vi "Emitter.Test.vi"() -> ()   [LabVIEW 2016]
panel:
  in  "input json string":string="{\"values\":\"test\"}"
  in  "exchange name":u16(ring) items=["requests", "alerts"]
  in  "routing key":string="broadcast"
  out "error out":errorcluster
  in  "error (in)":errorcluster
  in  "host name":string="higgsino.physics.ucsb.edu"
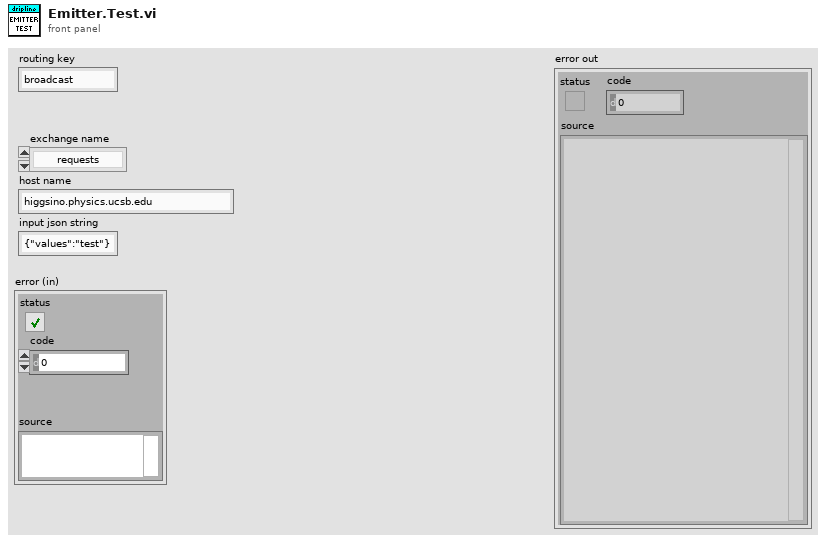
[diagram p1: front panel]
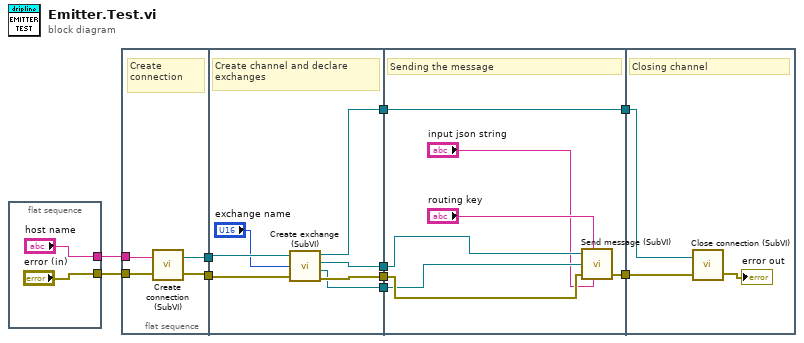
[diagram p0: block diagram]
diagram:
  n1 = flat-sequence {
    tunnel: ["error (in)"] -> w10
    tunnel: ["host name"] -> w9
    frame #0 {
    }
  }
  n2 = flat-sequence {
    tunnel: [w14] -> w8
    tunnel: [w15] -> w7
    tunnel: w9 -> [w16]
    tunnel: w10 -> [w13]
    tunnel: w8 -> [w23]
    tunnel: w7 -> [w22]
    tunnel: [w21] -> w6
    tunnel: [w20] -> w5
    tunnel: [w18] -> w2
    tunnel: [w17] -> w1
    tunnel: w6 -> [w27]
    tunnel: w5 -> [w30]
    tunnel: [w29] -> w4
    tunnel: [w28] -> w3
    tunnel: w2 -> [w28]
    tunnel: w1 -> [w26]
    tunnel: w4 -> [w33]
    tunnel: w3 -> [w32]
    frame #0 {
      # "Create connection"
      n3 = call "Create connection (SubVI).vi"("error in (no error)"=w13, "host name"=w16) -> ("error out"=w15:errorcluster, "Connection out"=w14:refnum<class "Connection.lvclass">)
    }
    frame #1 {
      # "Create channel and declare exchanges"
      n4 = call "Create exchange (SubVI).vi"("Connection in"=w23, "exchange name"="exchange name", "error in (no error)"=w22) -> ("Connection out"=w18:refnum<class "Connection.lvclass">, "Exchange.lvclass"=w20:refnum<class "Exchange.lvclass">, "Channel out"=w17:refnum<class "Channel.lvclass">, "error out"=w21:errorcluster)
    }
    frame #2 {
      # "Sending the message"
      n5 = call "Send message (SubVI).vi"("Exchange.lvclass"=w30, "target"="routing key", "Channel in"=w26, "error in (no error)"=w27, "body"="input json string") -> ("error out"=w29:errorcluster)  [unwired: 3 out]
    }
    frame #3 {
      # "Closing channel"
      n6 = call "Close connection (SubVI).vi"("error in (no error)"=w33, "Connection in"=w32) -> ("error out"=→"error out":errorcluster)  [unwired: 1 in]
    }
  }
